vi "探头恢复出厂.vi"(7 "校准参数":u16(ring) caption="校准参数：" items=["pH", "DO", "浊度", "电导率", "叶绿素a", "藻密度", "ORP", "DO2"], 8 "error in (no error)":errorcluster caption="错误输入（无错误）") -> (0 "error out":errorcluster caption="错误输出")   [LabVIEW 2016, in "斯坦道多参数.lvlib"]
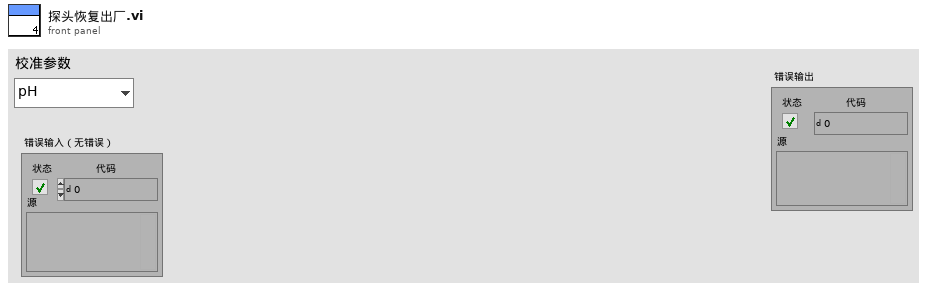
[diagram p1: front panel]
types:
  T1 = enum16{"null", "pH", "DO", "浊度", "电导率", "叶绿素a", "DO2"}
  T2 = enum16{"NULL", "pH", "Cond", "DO", "Turb", "ORP"}
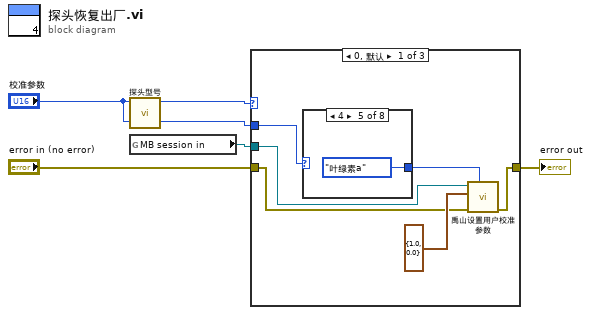
[diagram p0: block diagram]
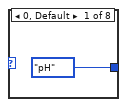
[diagram p2: hidden frame]
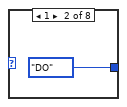
[diagram p3: hidden frame]
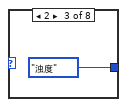
[diagram p4: hidden frame]
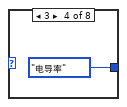
[diagram p5: hidden frame]
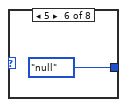
[diagram p6: hidden frame]
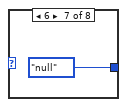
[diagram p7: hidden frame]
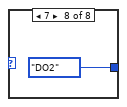
[diagram p8: hidden frame]
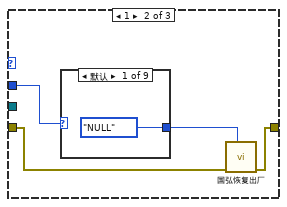
[diagram p9: hidden frame]
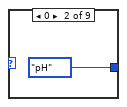
[diagram p10: hidden frame]
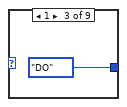
[diagram p11: hidden frame]
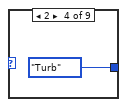
[diagram p12: hidden frame]
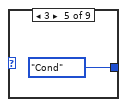
[diagram p13: hidden frame]
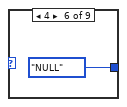
[diagram p14: hidden frame]
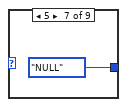
[diagram p15: hidden frame]
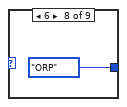
[diagram p16: hidden frame]
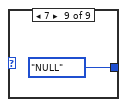
[diagram p17: hidden frame]
diagram:
  n1 = call "探头型号.vi"("校准参数"="校准参数") -> ("探头型号"=w5:u16)  [unwired: 8 in, 2 out]
  n2 = global read "多参数全局变量.vi" "MB session in"() -> (w1:refnum<class "MB_Master.lvclass">)
  n3 = case shown="0, 默认" w5 {
    tunnel: "校准参数" -> [w11 w23 _]
    tunnel: "error in (no error)" -> [w7 w21 w33]
    tunnel: [w6 w20 w33] -> w2
    tunnel: w1 -> [w8 _ _]
    frame 0, Default {
      n4 = case shown="4" w11 {
        tunnel: [T1."pH" ("探头") T1."DO" ("探头") T1."浊度" ("探头") T1."电导率" ("探头") T1."叶绿素a" ("探头") T1."null" ("探头") T1."null" ("探头") T1."DO2" ("探头")] -> w9
        frame 0, Default {
        }
        frame 1 {
        }
        frame 2 {
        }
        frame 3 {
        }
        frame 4 {
        }
        frame 5 {
        }
        frame 6 {
        }
        frame 7 {
        }
      }
      n5 = call "禹山设置用户校准参数.vi"("探头"=w9, "error in (no error)"=w7, "用户校准参数"=cluster{"K":sgl, "B":sgl} {"K"=1.0, "B"=0.0}, "MB session in"=w8) -> ("error out"=w6:errorcluster)  [unwired: 6 in, 1 out]
    }
    frame 1 {
      n6 = case shown="默认" w23 {
        tunnel: [T2."NULL" ("探头") T2."pH" ("探头") T2."DO" ("探头") T2."Turb" ("探头") T2."Cond" ("探头") T2."NULL" ("探头") T2."NULL" ("探头") T2."ORP" ("探头") T2."NULL" ("探头")] -> w22
        frame Default {
        }
        frame 0 {
        }
        frame 1 {
        }
        frame 2 {
        }
        frame 3 {
        }
        frame 4 {
        }
        frame 5 {
        }
        frame 6 {
        }
        frame 7 {
        }
      }
      n7 = call "国弘恢复出厂.vi"("探头"=w22, "error in (no error)"=w21) -> ("error out"=w20:errorcluster)  [unwired: 8 in, 1 out]
    }
    frame 2 {
    }
  }
  "error out" <- w2
